vi "ErrorInOut.vi"() -> ()   [LabVIEW 2017]
doc: "Places <B>Error in</B> and <B>Error out</B> controls with labels and captions formatted GPower-style.\n\nSteen Schmidt\nGPower\n16/11 2012"
panel:
  out "Error out":errorcluster
  in  "Error in":errorcluster caption="Error in (no error)"
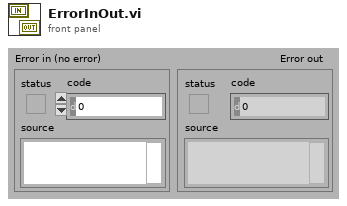
[diagram p1: front panel]
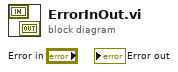
[diagram p0: block diagram]
diagram:
